vi "Launcher - top level VI.vi"() -> ()   [LabVIEW 2018]
doc: "Launches all ATM modules"
uses:
  Common/Common.lvlib
  Common/ctl/Stop all modules states--enum.ctl
  Controller/Controller.lvlib
  Error Handler/Error Handler.lvlib
  Display Console/Simulated/Display Console.lvlib
  Sensor Interface/Simulated/Sensor Interface.lvlib
  User Console/Simulated/User Console.lvlib
panel:
  in  "error in":errorcluster
  out "error out":errorcluster
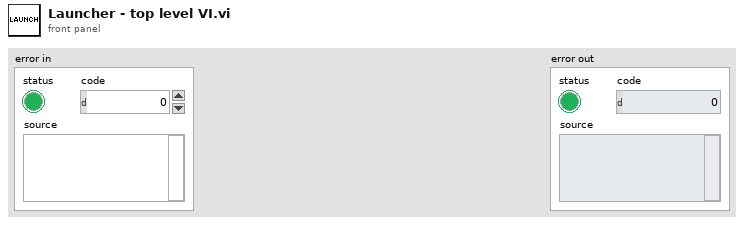
[diagram p1: front panel]
types:
  T1 = typedef "Common.lvlib/Stop all modules states--enum.ctl" = enum16{"Create", "Get", "Send 'Stop all' Message", "Destroy"}
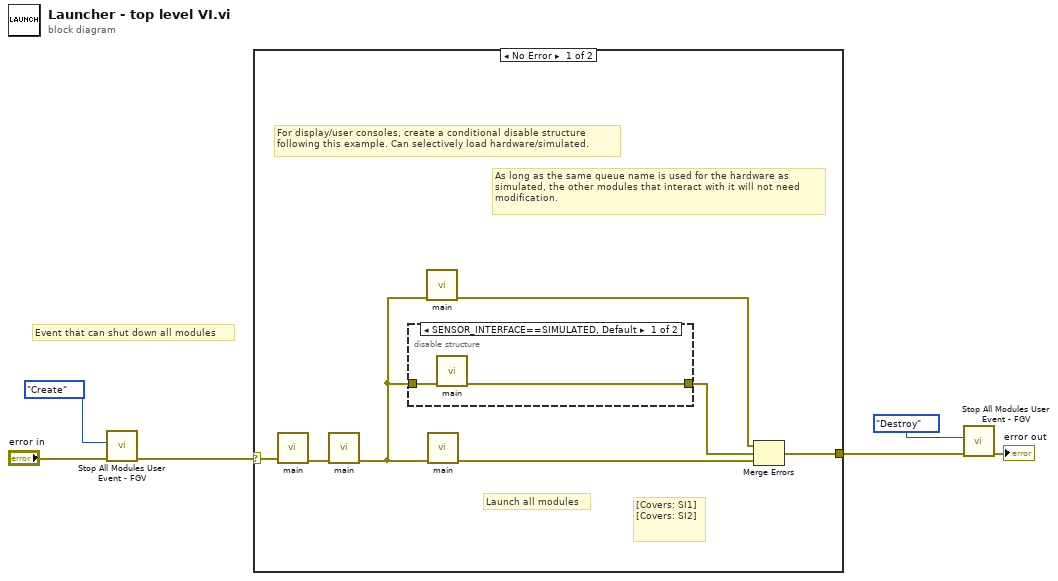
[diagram p0: block diagram]
diagram:
  # "Event that can shut down all modules"
  n1 = call "Stop All Modules User Event - FGV.vi"("error in"="error in", "Action"=Stop_all_modules_states--enum."Create") -> ("error out"=w4:errorcluster)  [unwired: 8 in, 1 out]
  n2 = case shown="No Error" w4 {
    selector: w4 -> [w13 w16]
    tunnel: [w7 w16] -> w3
    frame No Error {
      # "[Covers: SI1] \n[Covers: SI2]"
      # "As long as the same queue name is used for the hardware as\nsimulated, the other modules that interact with it will not need\nmodification."
      # "For display/user consoles, create a conditional disable structure\nfollowing this example. Can selectively load hardware/simulated."
      # "Launch all modules"
      n3 = call "main.vi"("Error in"=w13) -> ("error out"=w12:errorcluster)  [unwired: 10 in]
      n4 = call "main.vi"("Error in"=w12) -> ("error out"=w11:errorcluster)  [unwired: 10 in]
      n5 = disable-structure shown="SENSOR_INTERFACE==SIMULATED, Default" {
        disable-tunnel: w11 -> [w15 _]
        disable-tunnel: [w14 _] -> w9
        frame condition #0 (active) {
          n6 = call "main.vi"("Error in"=w15) -> ("error out"=w14:errorcluster)  [unwired: 10 in]
        }
        frame condition #1 {
          # "Insert replacement module here.\nUse simulated as a template"
        }
      }
      n7 = call "main.vi"("Error in"=w11) -> ("error out"=w10:errorcluster)  [unwired: 10 in]
      n8 = call "main.vi"("Error in"=w11) -> ("error out"=w8:errorcluster)  [unwired: 10 in]
      n9 = Merge Errors(w10, w9, w8) -> (w7:errorcluster)
    }
    frame Error {
    }
  }
  n10 = call "Stop All Modules User Event - FGV.vi"("error in"=w3, "Action"=Stop_all_modules_states--enum."Destroy") -> ("error out"=→"error out":errorcluster)  [unwired: 8 in, 1 out]
